vi "tdms_PDW_read.vi"() -> ()   [LabVIEW 2021]
doc: "This example demonstrates how to benchmark the streaming performance when you use the TDMS Advanced Asynchronous I/O functions to read data from a .tdms file. This VI measures the time it takes to continuously read data from a file and calculates the average data throughput in bytes/second."
uses:
  FPGA/PDW interpoter params.ctl
panel:
  in  "PDW interpoter params":T1={"Fs (Hz)"=200000000, "fft size "=4096, "F base (Hz)"=2000000000, "min AMP (dB)"=0.0, "PW low bar (fft cycle)"=0.0, "Pw high bar (fft cycle)"=7000.0, "lo likege removal (fft bin)"=-1, "max gap (fft cycle)"=0.0}
  out "Array":T2(array[cluster]) {"frequncy" format="%#_5p"; "PW" format="%#_3p"; "AMP" format="%#_3p"; "t end" format="%#_9g"}
  out "PW_resolotion":dbl format="%#_6p"
  out "frequncy resolotion":dbl format="%#_3p"
  out "time":dbl[](graph)
  out "mun of polses detections":i32
  in  "min amp":dbl format="%_3p"
  out "AMP":dbl[](graph)
  in  "Pw high bar":dbl=65535.0
  in  "PW low bar (# of tick)":dbl
  out "PW":dbl[](graph)
  out "frequncy":dbl[](graph)
  in  "F base":u32 format="%.0p"
  in  "Fs":u32=200000000 format="%.0p"
  in  "fft size":u32=4096
  in  "file path":path=path "C:/Users/NI/Documents/LabVIEW Data/streaming_test.tdms"
  # "TDMS file tester - receiver"
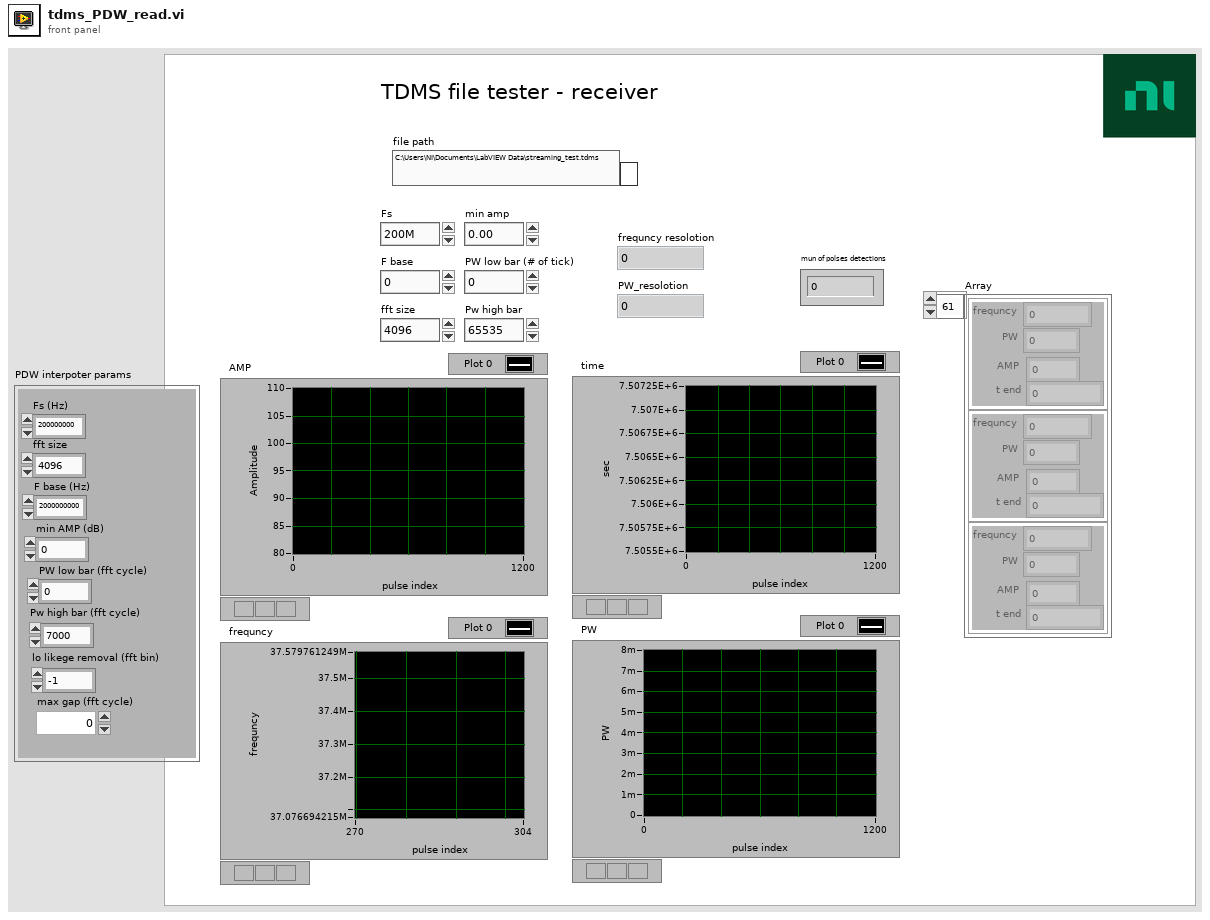
[diagram p1: front panel]
types:
  T1 = typedef "PDW interpoter params.ctl" = cluster{"Fs (Hz)":u32, "fft size ":u32, "F base (Hz)":u32, "min AMP (dB)":dbl, "PW low bar (fft cycle)":dbl, "Pw high bar (fft cycle)":dbl, "lo likege removal (fft bin)":i32, "max gap (fft cycle)":dbl}
  T2 = cluster{"frequncy":dbl, "PW":dbl, "AMP":dbl, "t end":dbl}[]
  T3 = enum16{"open", "open or create", "create or replace", "create", "open (read-only)"}
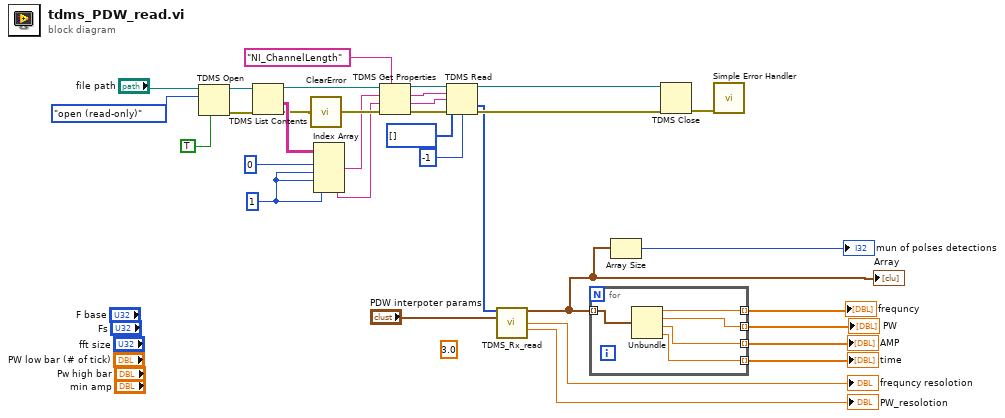
[diagram p0: block diagram]
diagram:
  (unwired) 3.0 ("max gap")
  w30 = 1 ("disabled index (col)")
  n1 = TDMS Open(6:TRUE ("disable buffering? (T)"), 10:T3."open (read-only)" ("Operation"), 11:"file path") -> (0:w27:errorcluster, 3:w26:refnum<k34>)  [unwired: 4 in]
  n2 = TDMS List Contents(4:w27, 7:w26) -> (0:w25:errorcluster, 1:w32:string[][], 3:w22:refnum<k34>)  [unwired: 1 in, 1 out]
  n3 = call <vilib>:"ClearError.vi"("error in (no error)"=w25) -> ("error out"=w29:errorcluster)
  n4 = Index Array(array=w32, index (row) #1=0 ("index (row)"), index (col) #1=w30, index (row) #2=w30, index (col) #2=w30) -> (element #1=w20:string, element #2=w19:string)
  n5 = TDMS Get Properties(7:"NI_ChannelLength" ("property name"), 8:w29, 9:w19, 10:w20, 11:w22) -> (0:w14:errorcluster, 1:w11:string, 2:w13:string, 3:w12:refnum<k34>)  [unwired: 1 in, 2 out]
  n6 = TDMS Read(0:w12, 2:i64 -1 ("count (-1: all)"), 5:w13, 7:w11, 11:w14, 12:u64[] []) -> (4:w8:refnum<k34>, 10:w9:u64[], 15:w10:errorcluster)  [unwired: 2 in, 3 out]
  n7 = call "TDMS_Rx_read.vi"("Array in"=w9, "PDW interpoter params"="PDW interpoter params") -> ("Array"=w7:cluster{dbl, dbl, "fixed-point":dbl, dbl}[], "frequncy resolotion"=→"frequncy resolotion":dbl, "PW_resolotion"=→"PW_resolotion":dbl)  [unwired: 11 in]
  "Array" <- w7
  n8 = for {
    tunnel: w7 -> [w38] mode=indexing
    tunnel: [w37] -> w17 mode=indexing
    tunnel: [w36] -> w16 mode=indexing
    tunnel: [w35] -> w15 mode=indexing
    tunnel: [w34] -> w4 mode=indexing
    n9 = Unbundle(w38) -> (w37:dbl, w36:dbl, "fixed-point"=w35:dbl, w34:dbl)
  }
  "frequncy" <- w17
  "PW" <- w16
  "AMP" <- w15
  "time" <- w4
  n10 = Array Size(array=w7) -> (size(s)=→"mun of polses detections":i32)
  n11 = TDMS Close(8:w10, 11:w8) -> (0:w5:errorcluster)  [unwired: 1 out]
  n12 = call <vilib>:"Simple Error Handler.vi"("error in (no error)"=w5) -> ()  [unwired: 1 in, 8 out]
